vi "brc_daq_get_last_error.vi"(0 "return_value":i32) -> (19 "error out":errorcluster)   [LabVIEW 2015, in "BRC-DAQ x86.lvlib"]
uses:
  BRC-DAQ x86.lvlib
  DLL/brc_daq_sdk.dll
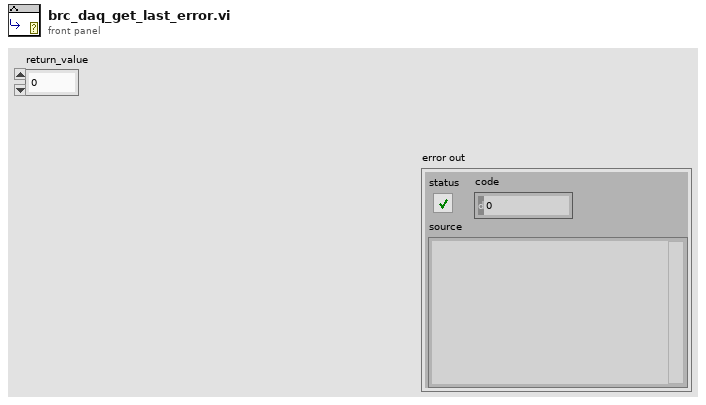
[diagram p1: front panel]
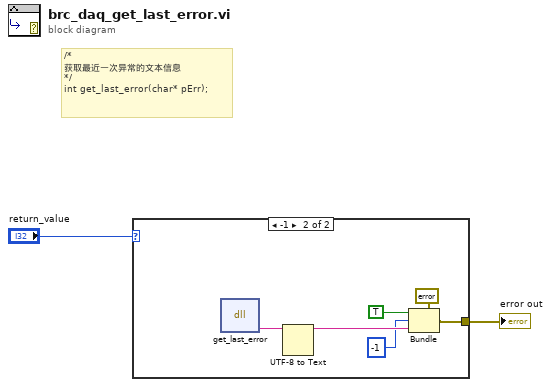
[diagram p0: block diagram]
diagram:
  # "/*\n获取最近一次异常的文本信息\n*/\nint get_last_error(char* pErr);"
  n1 = case shown="-1" "return_value" {
    tunnel: [_ w4] -> w2
    frame 0, Default {
    }
    frame -1 {
      n2 = dll-call lib="E:/01 BRC project/04BRC-daq/04 Drive/BRC-DAQ/DAQ-x86/DLL/brc_daq_sdk.dll" fn="get_last_error"() -> ("pErr"=w8:string)  [unwired: 5 in, 2 out]
      n3 = UTF-8 to Text(11:w8) -> (3:w6:string)  [unwired: 2 in, 1 out]
      n4 = Bundle(cluster=errorcluster {"status"=FALSE, "code"=0, "source"=""} ("error constant"), "status"=TRUE, "code"=-1, "source"=w6) -> (w4:errorcluster)
    }
  }
  "error out" <- w2
